vi "FTW-ERR-SerializeForLog.vi"(1 "error in":errorcluster) -> (0 "Serialized Error":string)   [LabVIEW 2014]
panel:
  # "Inputs"
  # "Outputs"
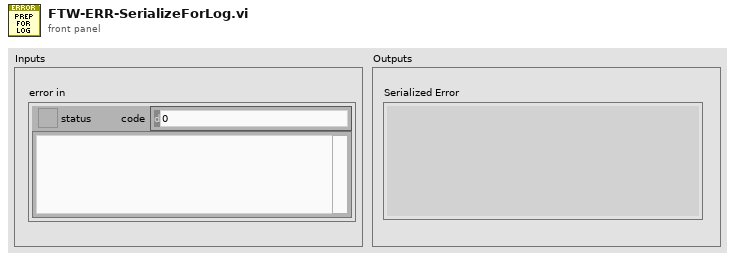
[diagram p1: front panel]
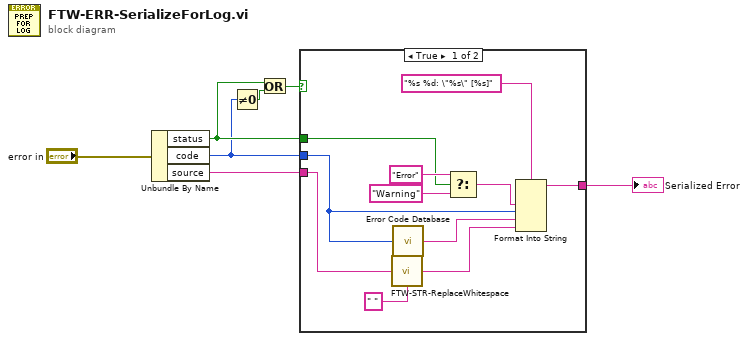
[diagram p0: block diagram]
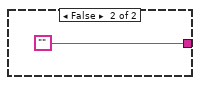
[diagram p2: hidden frame]
diagram:
  n1 = Unbundle By Name("error in") -> ("status"=w3:bool, "code"=w2:i32, "source"=w1:string)
  n2 = Not Equal To 0?(x=w2) -> (x != 0?=w4:bool)
  n3 = Or(x=w3, y=w4) -> (x .or. y?=w6:bool)
  n4 = case shown="True" w6 {
    tunnel: [w17 ""] -> w7
    tunnel: w3 -> [w12 _]
    tunnel: w2 -> [w10 _]
    tunnel: w1 -> [w16 _]
    frame True {
      n5 = call "FTW-STR-ReplaceWhitespace.vi"("Replace Spaces With..."=" ", "Input"=w16) -> ("Output"=w9:string)  [unwired: 2 in]
      n6 = call <vilib>:"Error Code Database.vi"("Error Code"=w10) -> ("Error Text"=w8:string)
      n7 = Select(t="Error", s=w12, f="Warning") -> (s? t:f=w13:string)
      n8 = Format Into String(format string="%s %d: \"%s\" [%s]", w13, w10, w8, w9) -> (resulting string=w17:string)  [unwired: 2 in, 1 out]
    }
    frame False {
    }
  }
  "Serialized Error" <- w7
